vi "ep_Check Fs Value.vi"(8 "error in (no error)":errorcluster, 11 "fundamental frequency [Hz]":dbl) -> (0 "error out":errorcluster)   [LabVIEW 2014, in "NI_EP_Motor Monitoring.lvlib"]
uses:
  <vilib>/addons/Electrical Power/Motor Monitoring/NI_EP_Motor Monitoring.lvlib
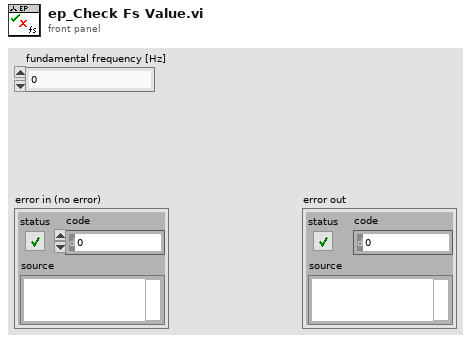
[diagram p1: front panel]
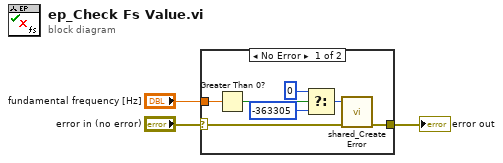
[diagram p0: block diagram]
diagram:
  n1 = case shown="No Error" "error in (no error)" {
    selector: "error in (no error)" -> [w5 w11]
    tunnel: [w10 w11] -> w3
    tunnel: "fundamental frequency [Hz]" -> [w4 _]
    frame No Error {
      n2 = Greater Than 0?(x=w4) -> (x > 0?=w9:bool)
      n3 = Select(t=0 ("error code (0)"), s=w9, f=-363305 ("error code (0)")) -> (s? t:f=w6:i32)
      n4 = call <vilib>:"shared_Create Error.vi"("error in (no error)"=w5, "error code (0)"=w6) -> ("error out"=w10:errorcluster)  [unwired: 9 in]
    }
    frame Error {
    }
  }
  "error out" <- w3
